vi "Open Session.vi"(8 "error in":errorcluster, 11 "Path":path) -> (0 "error out":errorcluster, 3 "Config Data":refnum<class "Config Data.lvclass">)   [LabVIEW 2015, in "Config Data.lvclass"]
uses:
  Config Data.lvclass
  Config Data.lvclass/Config Data.ctl
  <vilib>/Utility/config.llb/NI_LVConfig.lvlib
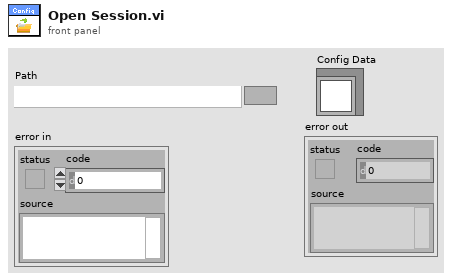
[diagram p1: front panel]
types:
  T1 = typedef "NI_LVConfig.lvlib/Config Data RefNum.ctl" = refnum<k1>
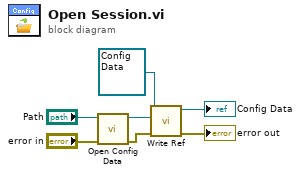
[diagram p0: block diagram]
diagram:
  n1 = call <vilib>:"Open Config Data.vi"("error in (no error)"="error in", "configuration file path"="Path") -> ("error out"=w3:errorcluster, "refnum"=w6:T1)  [unwired: 7 in, 1 out]
  n2 = call "Write Ref.vi"("error in (no error)"=w3, "config data"=w6, "Config Data in"=refnum<class "Config Data.lvclass"> refnum ("Config Data")) -> ("error out"=→"error out":errorcluster, "Config Data out"=→"Config Data":refnum<class "Config Data.lvclass">)  [unwired: 7 in]
